vi "Write Warm-Up Time.vi"(8 "error in (no error)":errorcluster, 10 "Warm-Up Time":dbl, 11 "1600 Card Actor in":refnum<class "1600 Card Actor.lvclass">) -> (0 "error out":errorcluster, 3 "1600 Card Actor out":refnum<class "1600 Card Actor.lvclass">)   [LabVIEW 2013, in "Universal Power Meter.lvlib" / "WT1600.lvlib" / "1600Card.lvlib" / "1600 Card Actor.lvclass"]
uses:
  1600 Card Actor.lvclass
  1600 Card Actor.lvclass/1600 Card Actor.ctl
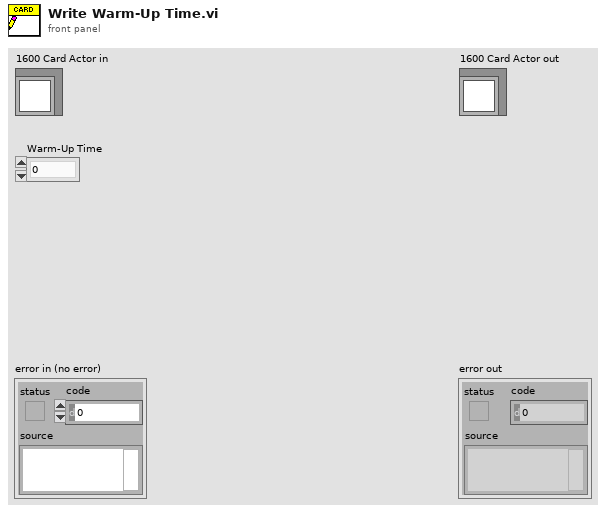
[diagram p1: front panel]
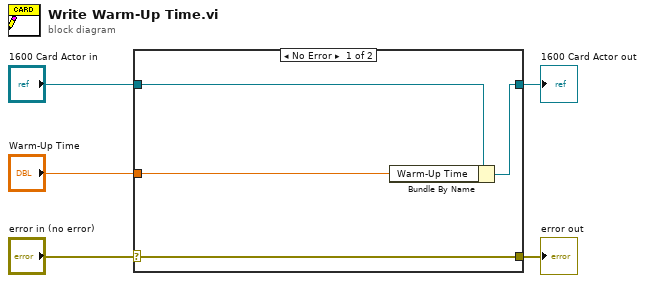
[diagram p0: block diagram]
diagram:
  n1 = case shown="No Error" "error in (no error)" {
    selector: "error in (no error)" -> [w9 w10]
    tunnel: [w9 w10] -> w4
    tunnel: [w7 w11] -> w2
    tunnel: "1600 Card Actor in" -> [w8 w11]
    tunnel: "Warm-Up Time" -> [w6 _]
    frame No Error {
      n2 = Bundle By Name(cluster=w8, "Warm-Up Time"=w6) -> (w7:refnum<class "1600 Card Actor.lvclass">)
    }
    frame Error {
    }
  }
  "error out" <- w4
  "1600 Card Actor out" <- w2
